vi "Zaber Expert - Change Timeout.vi"() -> ()   [LabVIEW 2015]
doc: "Connect your Zaber device to power and a serial port, then select the serial port below. Click the Run arrow above, and this will send an Echo\ncommand to device number 1 to make sure it's connected, then send a home command.\nIf you disconnect the power and then Click the Run arrow, you'll get a timeout error. If you run one of the beginner examples with disconnected power, it just waits for a response forever and never finishes.\nTimeouts are disabled by default because some movement commands can take a long time to execute. Most will finish in a few seconds, but a large device executing a slow move could take hours.\nHowever, timeouts can be useful for detecting things like a disconnected device. This shows you how to set the timeout before a command, and then set it back to its original value.\nAlthough movement commands can vary widely in how long they take to complete, any command that changes or reads a setting will respond in less than a second."
uses:
  ZaberTSeries.lvlib
  Public/Utility/Request.ctl
panel:
  in  "VISA resource name":refnum<visa-resource-name>
  # "Connect your Zaber device to power and a serial port, then select the\nserial port below. Click the Run arrow above, and this will send an Echo\ncommand to device number 1 to make sure it's connected, then send a\nhome command.\nIf you disconnect the power and then Click the Run arrow, you'll get a\ntimeout error. If you run one of the beginner examples with disconnected\npower, it just waits for a response forever and never finishes. \nType Ctrl-E to see how the block diagram is wired."
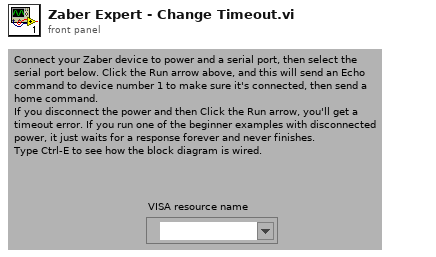
[diagram p1: front panel]
types:
  T1 = typedef "ZaberTSeries.lvlib/Request.ctl" = cluster{"Device Number":u8, "Command":u8, "Data":i32, "Response Count":i32}
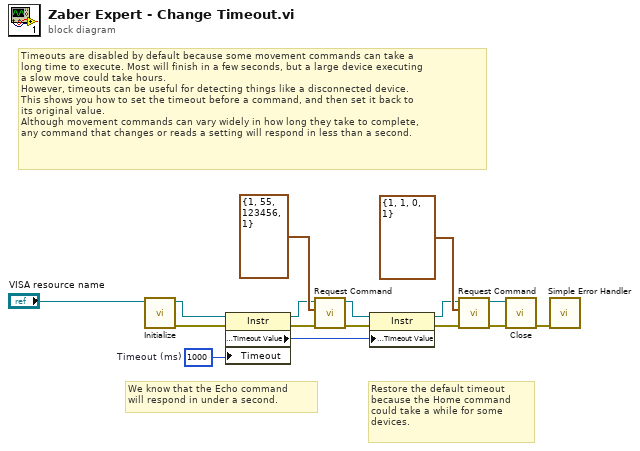
[diagram p0: block diagram]
diagram:
  w8 = u32 1000  # Timeout (ms)
  # "Timeouts are disabled by default because some movement commands can take a\nlong time to execute. Most will finish in a few seconds, but a large device executing\na slow move could take hours.\nHowever, timeouts can be useful for detecting things like a disconnected device.\nThis shows you how to set the timeout before a command, and then set it back to\nits original value.\nAlthough movement commands can vary widely in how long they take to complete,\nany command that changes or reads a setting will respond in less than a second."
  # "Restore the default timeout\nbecause the Home command\ncould take a while for some\ndevices."
  # "We know that the Echo command\nwill respond in under a second."
  n1 = call "Initialize.vi"("VISA resource name"="VISA resource name") -> ("error out"=w9:errorcluster, "VISA resource name out"=w10:refnum<visa-resource-name>)  [unwired: 8 in, 1 out]
  n2 = property class="Instr"(reference=w10, error in=w9, "Timeout"=w8) -> (reference out=w7:refnum<visa-resource-name>, error out=w6:errorcluster, "General Settings:Timeout Value"=w1:u32)
  n3 = call "Request Command.vi"("error in (no error)"=w6, "Request"=T1 {"Device Number"=1, "Command"=55, "Data"=123456, "Response Count"=1}, "VISA resource name"=w7) -> ("error out"=w4:errorcluster, "VISA resource name out"=w5:refnum<visa-resource-name>)  [unwired: 5 in, 2 out]
  n4 = property class="Instr"(reference=w5, error in=w4, "General Settings:Timeout Value"=w1) -> (reference out=w3:refnum<visa-resource-name>, error out=w2:errorcluster)
  n5 = call "Request Command.vi"("error in (no error)"=w2, "Request"=T1 {"Device Number"=1, "Command"=1, "Data"=0, "Response Count"=1}, "VISA resource name"=w3) -> ("error out"=w12:errorcluster, "VISA resource name out"=w13:refnum<visa-resource-name>)  [unwired: 5 in, 2 out]
  n6 = call "Close.vi"("error in (no error)"=w12, "VISA resource name"=w13) -> ("error out"=w15:errorcluster)  [unwired: 8 in, 1 out]
  n7 = call <vilib>:"Simple Error Handler.vi"("error in (no error)"=w15) -> ()  [unwired: 4 in, 5 out]
